vi "p-p0 and normaiize .vi"(0 "po file path":path, 1 "length":dbl[](array[numeric]), 2 "power":dbl[](array[numeric])) -> (3 "SPR wave length(nm)":string, 4 "SPR efficiency":string, 5 "length 2":dbl[](array[numeric]), 6 "normallize power":dbl[](array[numeric]))   [LabVIEW 2019]
uses:
  <vilib>/Utility/file.llb/Read From Spreadsheet File (string).vi
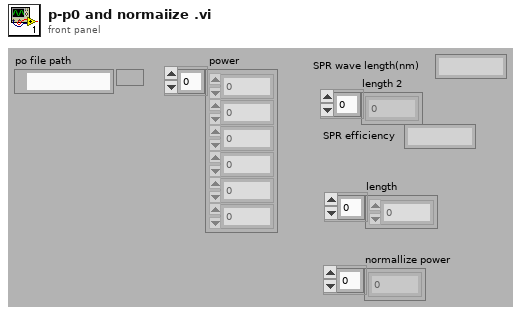
[diagram p1: front panel]
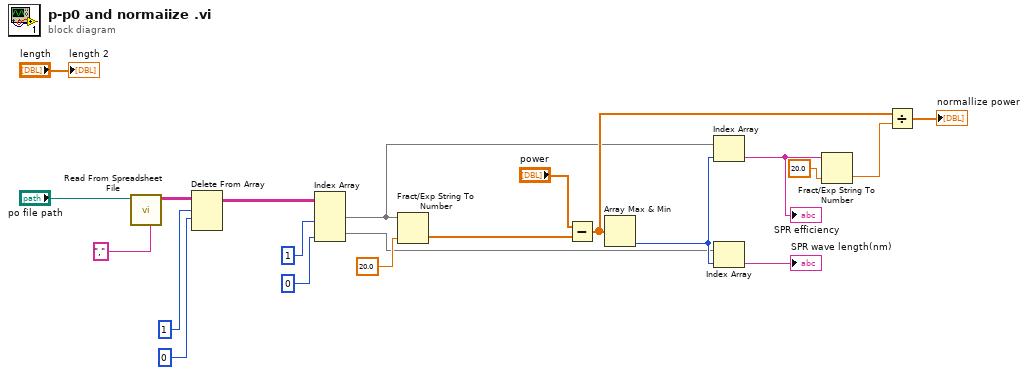
[diagram p0: block diagram]
diagram:
  n1 = call-poly <vilib>:"Read From Spreadsheet File.vi"("delimiter (\\t)"="," ("delimiter (\\t)"), "file path (dialog if empty)"="po file path") -> ("all rows"=w12:string[][])  [unwired: 3 in, 6 out]
  n2 = Delete From Array "Delete From Array"(array=w12, length=1, index (row)=0 ("index")) -> (array with subset deleted=w14:string[][])  [unwired: 1 in, 1 out]
  n3 = Index Array "Index Array"(array=w14, index (col) #1=1 ("disabled index (col)"), index (col) #2=0 ("index (col)")) -> (element #1=w3:string[], element #2=w2:string[])  [unwired: 2 in]
  n4 = Fract/Exp String To Number(string=w3, default (0 dbl)=20.0 ("default (0 DBL)")) -> (number=w19:dbl[])  [unwired: 3 out]
  n5 = Subtract(x="power", y=w19) -> (x-y=w18:dbl[])
  n6 = Array Max & Min(array=w18) -> (min index (indices)=w4:i32)  [unwired: 3 out]
  n7 = Index Array "Index Array"(array=w3, index=w4) -> (element=w1:string)
  "SPR efficiency" <- w1
  n8 = Index Array "Index Array"(array=w2, index=w4) -> (element=→"SPR wave length(nm)":string)
  n9 = Fract/Exp String To Number(string=w1, default (0 dbl)=20.0 ("default (0 DBL)")) -> (number=w17:dbl)  [unwired: 3 out]
  n10 = Divide(x=w18, y=w17) -> (x/y=→"normallize power":dbl[])
  "length 2" <- "length"
